vi "example_3_4_a.vi"() -> ()   [LabVIEW 2018]
panel:
  in  "Capture":bool
  in  "stop":bool
  out "Intensity":i16
  out "Blue":i16
  out "Green":i16
  out "Red":i16
  in  "Fiber number":u16=1 min=1 max=20
  # "NOTE: remember plug the Led Analyser\nbefore run LabVIEW and to change the\nVISA resource name in the schematic,\notherwise the application will not work."
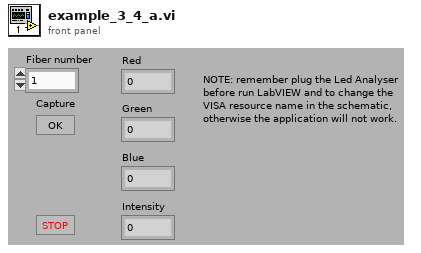
[diagram p1: front panel]
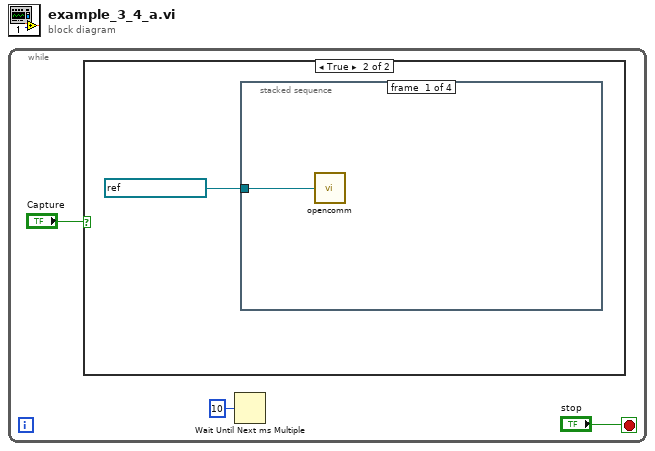
[diagram p0: block diagram]
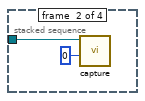
[diagram p3: hidden frame]
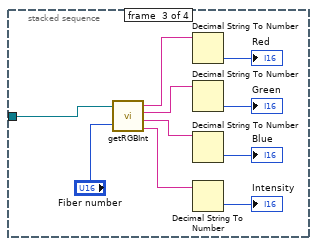
[diagram p4: hidden frame]
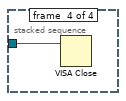
[diagram p5: hidden frame]
diagram:
  n1 = while {
    stop <- "stop" stop-if-true
    n2 = case shown="True" "Capture" {
      frame False {
      }
      frame True {
        n3 = stacked-sequence {
          tunnel: refnum<visa-resource-name> "ASRL20::INSTR" ("VISA resource name") -> [w5 w6 w8 w18]
          frame #0 {
            n4 = call "opencomm.vi"("VISA resource name"=w5) -> ()  [unwired: 2 out]
          }
          frame #1 {
            n5 = call "capture.vi"("Capture Range"=0 ("Capture Type"), "VISA resource name"=w6) -> ()  [unwired: 2 in, 2 out]
          }
          frame #2 {
            n6 = call "getRGBInt.vi"("VISA resource name"=w8, "Fiber Num"="Fiber number") -> ("R"=w12:string, "G"=w11:string, "B"=w10:string, "INT"=w9:string)
            n7 = Decimal String To Number(string=w12) -> (number=→"Red":i32)  [unwired: 2 in, 1 out]
            n8 = Decimal String To Number(string=w11) -> (number=→"Green":i32)  [unwired: 2 in, 1 out]
            n9 = Decimal String To Number(string=w10) -> (number=→"Blue":i32)  [unwired: 2 in, 1 out]
            n10 = Decimal String To Number(string=w9) -> (number=→"Intensity":i32)  [unwired: 2 in, 1 out]
          }
          frame #3 {
            n11 = VISA Close(VISA resource name=w18) -> ()  [unwired: 1 in, 1 out]
          }
        }
      }
    }
    n12 = Wait Until Next ms Multiple(millisecond multiple=u32 10) -> ()  [unwired: 1 out]
  }
